vi "getFPGAReadTimeout.vi"(11 "Modbus in":refnum<class "Modbus.lvclass">) -> (2 "FPGAReadTimeout":i32=1, 3 "Modbus out":refnum<class "Modbus.lvclass">)   [LabVIEW 2015, in "Modbus.lvclass"]
uses:
  Modbus.lvclass
  Modbus.lvclass/Modbus.ctl
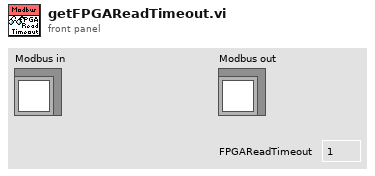
[diagram p1: front panel]
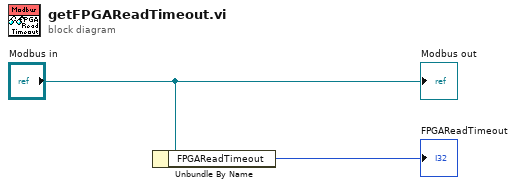
[diagram p0: block diagram]
diagram:
  n1 = Unbundle By Name("Modbus in") -> ("FPGAReadTimeout"=→"FPGAReadTimeout":i32)
  "Modbus out" <- "Modbus in"
